vi "02-Termometro.vi"() -> ()   [LabVIEW 2014]
panel:
  out "Thermometer":dbl(slide) scale=0.0..100.0
  in  "Temp Scale":bool
  # "Deg C"
  # "Deg F"
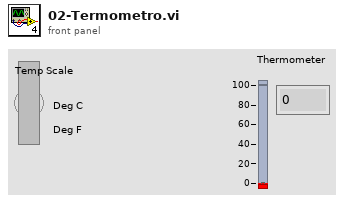
[diagram p1: front panel]
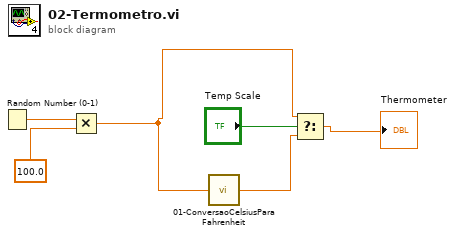
[diagram p0: block diagram]
diagram:
  n1 = Random Number (0-1)() -> (number: 0 to 1=w6:dbl)
  n2 = Multiply(x=w6, y=100.0 ("x*y")) -> (x*y=w1:dbl)
  n3 = call "01-ConversaoCelsiusParaFahrenheit.vi"("Deg C"=w1) -> ("Deg F"=w2:dbl)
  n4 = Select(t=w1, s="Temp Scale", f=w2) -> (s? t:f=→"Thermometer":dbl)
